vi "computeTorque.vi"(0 "X":dbl, 5 "Y":dbl, 7 "TrialParams":T2, 9 "MvmtHistory":T1, 11 "error in":errorcluster, 12 "Jt":dbl[][](array[numeric])) -> (4 "mvmtOver":bool, 6 "error out":errorcluster, 8 "MvmtHistoryOut":T1, 10 "Torque 1":i16, 15 "Torque 2":i16)   [LabVIEW 2019]
uses:
  MvmtHistory.ctl
  TrialParams.ctl
  trial type.ctl
  <vilib>/imath/engines/lvmath2/RunTimeEngine/ArithmeticOperatorToken/NIMS_ArithmeticOperator_multmx(M,CV)-internal.vi
  <instcachedir>/0/NIMS_ArithmeticOperator_multmx(M,CV)-internal_2C55777844884EEDB828A940D397C7D0.lvgen/NIMS_ArithmeticOperator_multmx(M,CV)-internal_2C55777844884EEDB828A940D397C7D0_001.vi
  <vilib>/imathl/engines/lvmath/Functions/Error Handling/Create Error.vi
  <vilib>/imath/engines/lvmath2/RunTimeEngine/IndexRead/NIMS V(S).vi
  <instcachedir>/0/NIMS V(S)_0488751826AF41519A22953C041130DC.lvgen/NIMS V(S)_0488751826AF41519A22953C041130DC_000.vi
  <vilib>/imath/engines/lvmath2/RunTimeEngine/IndexReplace/NIMS V($)=S.vi
  <instcachedir>/0/NIMS V($)=S_C017B4DE03EF471E928F9C524123803A.lvgen/NIMS V($)=S_C017B4DE03EF471E928F9C524123803A_000.vi
  <vilib>/imath/engines/lvmath/Functions/Error Handling/MergeErrorsWrapper.vi
  <vilib>/imath/engines/lvmath2/RunTimeEngine/VariableToken/NIMS_VariableToken_CondDefined.vi
  <instcachedir>/0/NIMS_VariableToken_CondDefined_30C3C94EAC01413DA882E848DEC89944.lvgen/NIMS_VariableToken_CondDefined_30C3C94EAC01413DA882E848DEC89944_001.vi
  <vilib>/imath/engines/lvmath2/RunTimeEngine/ErrorHandling/NIMS_Create Error From Enums.vi
  <vilib>/imath/engines/lvmath2/RunTimeEngine/IndexReplace/NIMS V(S)=S.vi
  <instcachedir>/0/NIMS V(S)=S_BD5C8CB81B6E4D99B8C0034EA1BEE55D.lvgen/NIMS V(S)=S_BD5C8CB81B6E4D99B8C0034EA1BEE55D_000.vi
  <vilib>/imath/engines/lvmath2/RunTimeEngine/ArithmeticOperatorToken/NIMS_ArithmeticOperator_multmx(M,CV).vi
  <instcachedir>/0/NIMS_ArithmeticOperator_multmx(M,CV)_1D61EED49E1847F3B05DBB8EDD2FBF8F.lvgen/NIMS_ArithmeticOperator_multmx(M,CV)_1D61EED49E1847F3B05DBB8EDD2FBF8F_000.vi
  <vilib>/imath/engines/lvmath2/RunTimeEngine/IndexRead/NIMS M(S).vi
  <instcachedir>/0/NIMS M(S)_B826C018497E4940AE96BD27B540B6FB.lvgen/NIMS M(S)_B826C018497E4940AE96BD27B540B6FB_000.vi
  <vilib>/imath/engines/lvmath2/RunTimeEngine/IndexRead/NIMS V(R2).vi
  <instcachedir>/0/NIMS V(R2)_C76619605A0E4E9F8B2FA9389712AC47.lvgen/NIMS V(R2)_C76619605A0E4E9F8B2FA9389712AC47_000.vi
  <vilib>/imath/engines/lvmath2/RunTimeEngine/NodeEndStatement/NIMS_NodeEndStatement_Output.vi
  <instcachedir>/0/NIMS_NodeEndStatement_Output_53EC0D466D134D7ABD903AC30B43404B.lvgen/NIMS_NodeEndStatement_Output_53EC0D466D134D7ABD903AC30B43404B_010.vi
  <instcachedir>/0/NIMS_NodeEndStatement_Output_53EC0D466D134D7ABD903AC30B43404B.lvgen/NIMS_NodeEndStatement_Output_53EC0D466D134D7ABD903AC30B43404B_001.vi
  <instcachedir>/0/NIMS_NodeEndStatement_Output_53EC0D466D134D7ABD903AC30B43404B.lvgen/NIMS_NodeEndStatement_Output_53EC0D466D134D7ABD903AC30B43404B_005.vi
  <vilib>/imath/engines/lvmath2/RunTimeEngine/ErrorHandling/NIMS_Finalize Error.vi
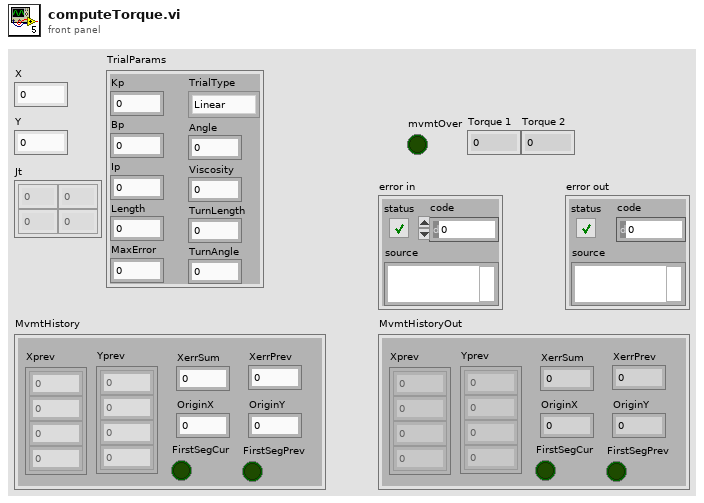
[diagram p1: front panel]
types:
  T1 = typedef "MvmtHistory.ctl" = cluster{"Xprev":dbl[], "Yprev":dbl[], "XerrSum":dbl, "XerrPrev":dbl, "OriginX":dbl, "OriginY":dbl, "FirstSegCur":bool, "FirstSegPrev":bool}
  T2 = typedef "TrialParams.ctl" = cluster{"Kp":dbl, "Bp":dbl, "Ip":dbl, "TrialType":T3, "Angle":dbl, "Viscosity":dbl, "Length":dbl, "MaxError":dbl, "TurnLength":dbl, "TurnAngle":dbl}
  T3 = typedef "trial type.ctl" = enum8{"Linear", "2D aiming", "Two-part"}
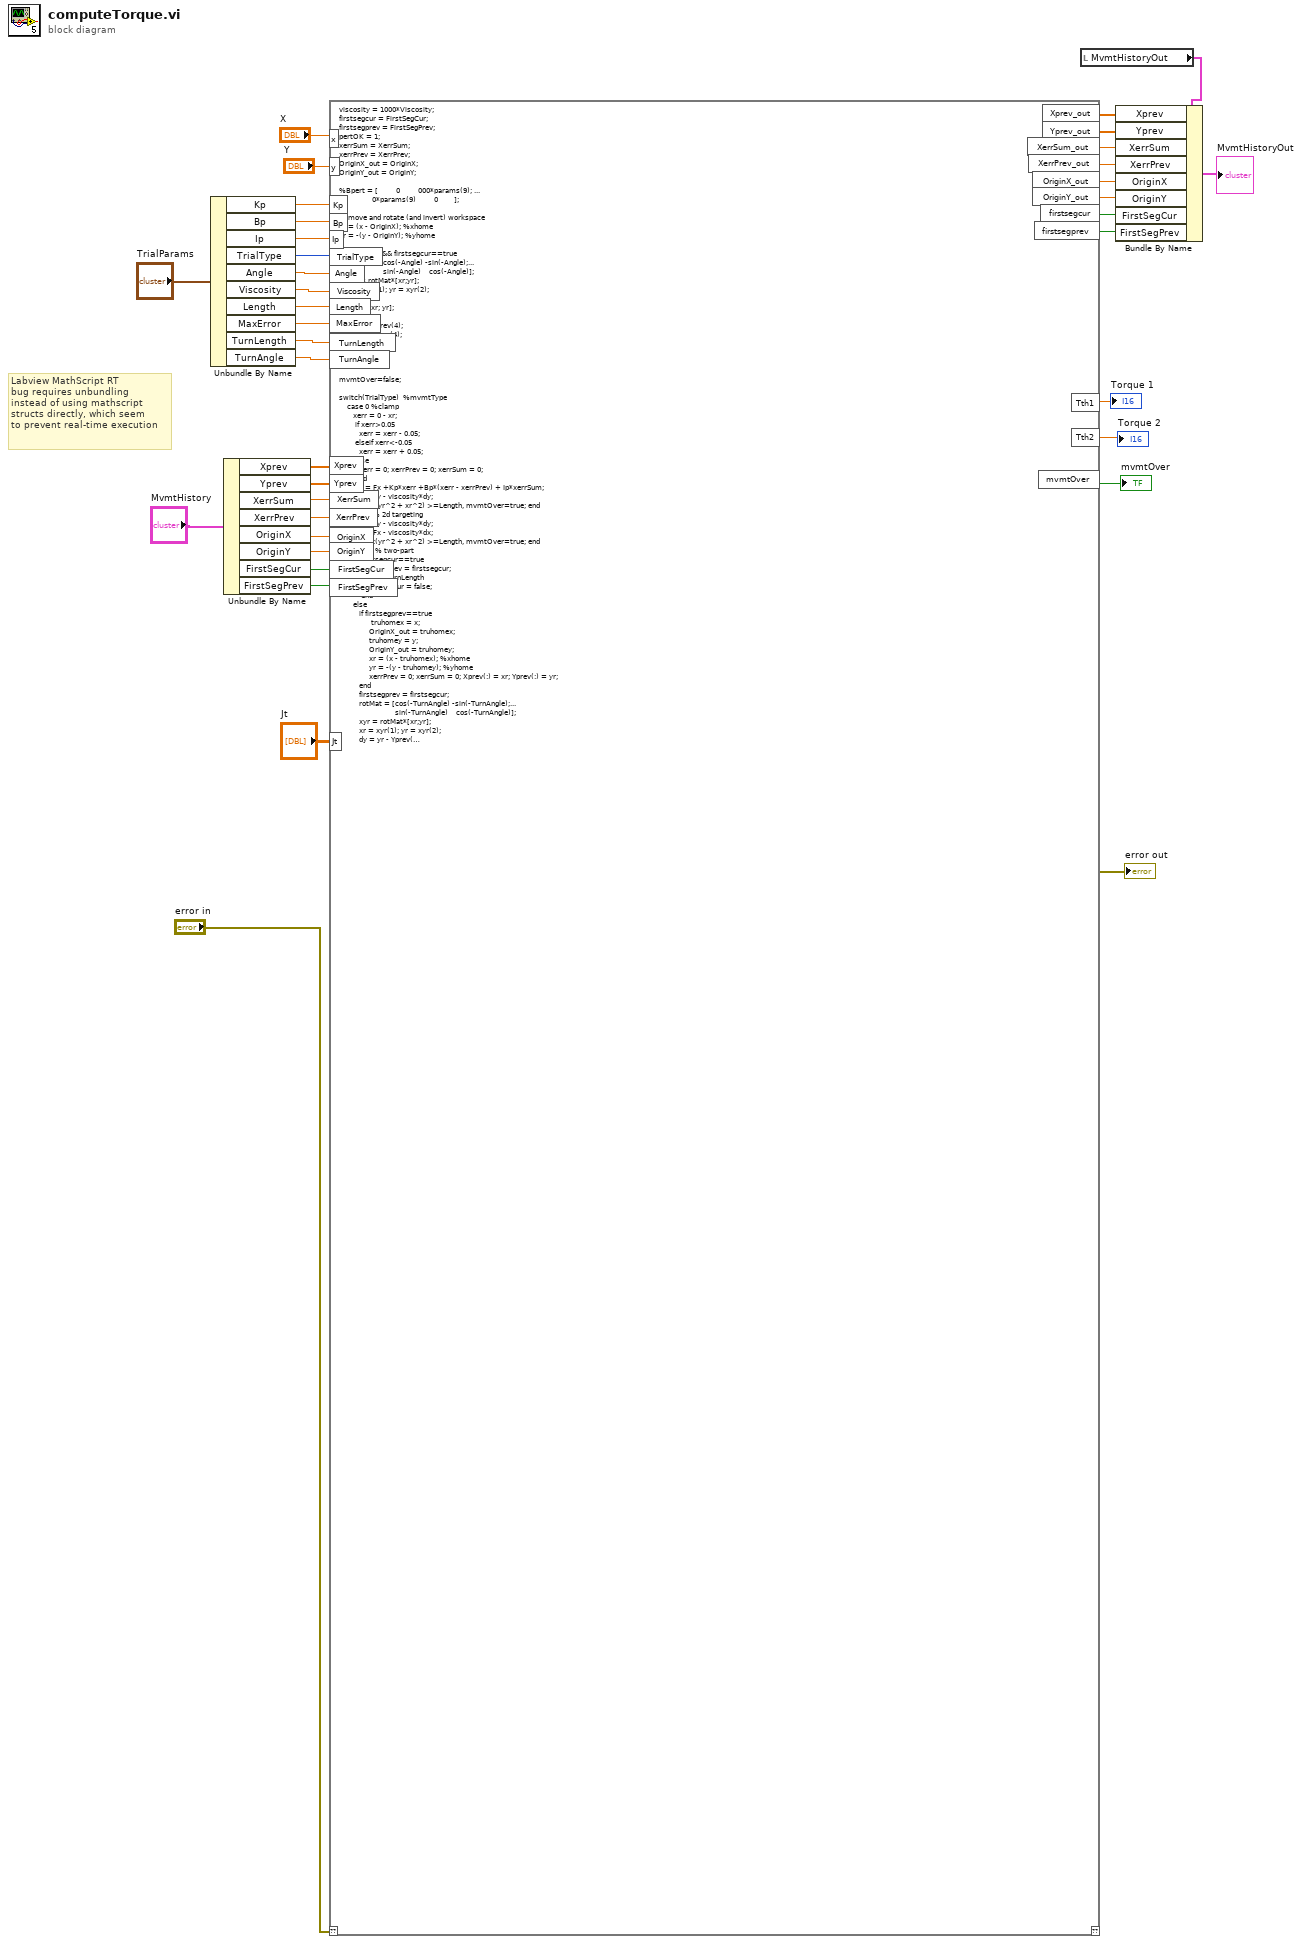
[diagram p0: block diagram]
diagram:
  # "Labview MathScript RT\nbug requires unbundling\ninstead of using mathscript\nstructs directly, which seem\nto prevent real-time execution"
  n1 = Unbundle By Name("TrialParams") -> ("Kp"=w18:dbl, "Bp"=w17:dbl, "Ip"=w16:dbl, "TrialType"=w19:T3, "Angle"=w22:dbl, "Viscosity"=w29:dbl, "Length"=w15:dbl, "MaxError"=w14:dbl, "TurnLength"=w13:dbl, "TurnAngle"=w12:dbl)
  n2 = Unbundle By Name("MvmtHistory") -> ("Xprev"=w20:dbl[], "Yprev"=w21:dbl[], "XerrSum"=w26:dbl, "XerrPrev"=w25:dbl, "OriginX"=w24:dbl, "OriginY"=w23:dbl, "FirstSegCur"=w28:bool, "FirstSegPrev"=w27:bool)
  n3 = mathscript code="viscosity = 1000*Viscosity;\nfirstsegcur = FirstSegCur;\nfirstsegprev = FirstSegPrev;\npertOK = 1;\nxerrSum = XerrSum;\nxerrPrev = XerrPrev;\nOriginX_out = OriginX;\nOriginY_out = OriginY;\n\n%Bpert = [         0         000*params(9); ...\n%             0*params(9)         0        ];\n\n% move and rotate (and invert) workspace\nxr = (x - OriginX); %xhome\nyr = -(y - OriginY); %yhome\n\nif Angle~=0 && firstsegcur==true\n    rotMat = [cos(-Angle) -sin(-Angle);...\n                      sin(-Angle)    cos(-Angle)];\n    xyr = rotMat*[xr;yr];\n\t   xr = xyr(1); yr = xyr(2);\nelse\n   \txyr = [xr; yr];\nend\ndx = xr - Xprev(4);\ndy = yr - Yprev(4);\nFx = 0;\nFy = 0;\nxerr = 0;\n \nmvmtOver=false; \n\nswitch(TrialType)\t %mvmtType\n    case 0 %clamp\n       xerr = 0 - xr;\n        if xerr>0.05\n          xerr = xerr - 0.05;\n        elseif xerr<-0.05\n          xerr = xerr + 0.05;\n        else\n          xerr = 0; xerrPrev = 0; xerrSum = 0;\n        end\n        Fx = Fx +Kp*xerr +Bp*(xerr - xerrPrev) + Ip*xerrSum;\n        Fy = Fy - viscosity*dy;\n        if sqrt(yr^2 + xr^2) >=Length, mvmtOver=true; end\n     case 1 % 2d targeting\n        Fy = Fy - viscosity*dy;\n        Fx = Fx - viscosity*dx;\n        if sqrt(yr^2 + xr^2) >=Length, mvmtOver=true; end\n     case  2 % two-part\n     \t\t\tif firstsegcur==true\n           firstsegprev = firstsegcur;\n       \t\t\t\tif yr>=TurnLength\n\t\t\t         \t\tfirstsegcur = false;\n    \t   \t\t\tend\n\t    \t\telse\n          if firstsegprev==true\n                truhomex = x;\n               OriginX_out = truhomex;\n               truhomey = y;\n               OriginY_out = truhomey;\n               xr = (x - truhomex); %xhome\n               yr = -(y - truhomey); %yhome\n               xerrPrev = 0; xerrSum = 0; Xprev(:) = xr; Yprev(:) = yr;\n          end\n          firstsegprev = firstsegcur;\n\t\t\t\t\t     rotMat = [cos(-TurnAngle) -sin(-TurnAngle);...\n                       \t\t\t\t\tsin(-TurnAngle)    cos(-TurnAngle)];\n     \t\t\t\t\txyr = rotMat*[xr;yr];\n          xr = xyr(1); yr = xyr(2);\n          dy = yr - Yprev(4);\n       \t\t\tif firstsegprev==false && yr >= TurnLength\n                mvmtOver=true; \n           end\n           if MaxError~=0 && ~firstsegcur && yr <= -MaxError\n               mvmtOver = true;\n           end\n    \t\t\tend\n    \t\t\txerr = 0 - xr;\n    \t\t\tif xerr>.05\n      \t\t\t\txerr = xerr - 0.05;\n    \t\t\telseif xerr<-.05\n      \t\t\t\txerr = xerr + 0.05;\n    \t\t\telse\n      \t\t\t\txerr = 0; xerrPrev = 0; xerrSum = 0;\n    \t\t\tend\n       Fx = Fx +Kp*xerr +Bp*(xerr - xerrPrev) +Ip*xerrSum;\n       Fy = Fy - viscosity*dy;           \nend\n% no pulling\nif yr<-0.7 && (firstsegcur==true || (firstsegcur==false && TrialType==2))\n    %if dy>-0.01, dy = 0; end\n    Fy = Fy - Kp/5*(yr+.7)  - Bp/5*(yr - Yprev(4));\nend\n% invert (transpose) rotation\nif (Angle~=0 && firstsegcur==true) || (TurnAngle~=0 && firstsegcur==false && firstsegprev==false)\n    Fxy = rotMat'*[Fx; Fy];\nelse\n    Fxy = [Fx; Fy];\nend\n\n% go back to upside down\nFxy(2) = -Fxy(2);\n% joint torques\nT = Jt*Fxy;\n% motor current = (torque/torqueconstant + no-load current)/quantization\n%I = T*27.8552 + 10.1*sign(T);\nTth1 = T(1); Tth2 = T(2);\nif mvmtOver\n    Tth1 = 0; Tth2 = 0;\nend\nXprev_out = [xr Xprev(1:3)];\nYprev_out = [yr Yprev(1:3)];\nxerrSum = xerrSum + xerr;\nif xerrSum > 0.5\n    xerrSum = 0.5;\nelseif xerrSum < -0.5\n    xerrSum = -0.5;\nend\nXerrPrev_out = xerr;\nXerrSum_out = xerrSum;"("??"="error in", "x"="X", "y"="Y", "Jt"="Jt", "Viscosity"=w29, "FirstSegCur"=w28, "FirstSegPrev"=w27, "XerrSum"=w26, "XerrPrev"=w25, "OriginX"=w24, "OriginY"=w23, "Angle"=w22, "Xprev"=w20, "Yprev"=w21, "TrialType"=w19, "Kp"=w18, "Bp"=w17, "Ip"=w16, "Length"=w15, "MaxError"=w14, "TurnLength"=w13, "TurnAngle"=w12) -> ("??"=→"error out":errorcluster, "Tth1"=→"Torque 1":dbl, "Tth2"=→"Torque 2":dbl, "mvmtOver"=→"mvmtOver":bool, "Xprev_out"=w10:dbl[], "Yprev_out"=w9:dbl[], "XerrSum_out"=w8:dbl, "XerrPrev_out"=w7:dbl, "OriginX_out"=w6:dbl, "OriginY_out"=w5:dbl, "firstsegcur"=w4:bool, "firstsegprev"=w3:bool)
  n4 = local read "MvmtHistoryOut"() -> (w2:T1)
  n5 = Bundle By Name(cluster=w2, "Xprev"=w10, "Yprev"=w9, "XerrSum"=w8, "XerrPrev"=w7, "OriginX"=w6, "OriginY"=w5, "FirstSegCur"=w4, "FirstSegPrev"=w3) -> (→"MvmtHistoryOut":T1)
